vi "KGN Set Concentrations.vi"(6 "Set Values Cluster":T2(array[cluster]), 7 "scaling":dbl, 8 "Fehler (Eingang, kein Fehler)":errorcluster, 9 "Info Cluster":T1, 10 "VISA-Referenz (Eingang)":refnum<visa-resource-name>, 11 "device (Eingang)":u32) -> (0 "Fehler (Ausgang)":errorcluster, 1 "Info Cluster out":T1, 2 "VISA-Referenz (Ausgang)":refnum<visa-resource-name>, 3 "dup device (Ausgang)":u32, 4 "Kommandos gesendet":string)   [LabVIEW 2020, in "Linearisierung v2.lvlib" / "Gasteiler.lvlib" / "HovaCAL_Interface.lvlib" / "KGN.lvlib" / "KGN GUI Set.lvlib"]
uses:
  KGN GUI Set.lvlib
  Controls/Info Cluster.ctl
  set/set.lvlib
  Controls/Controls.lvlib
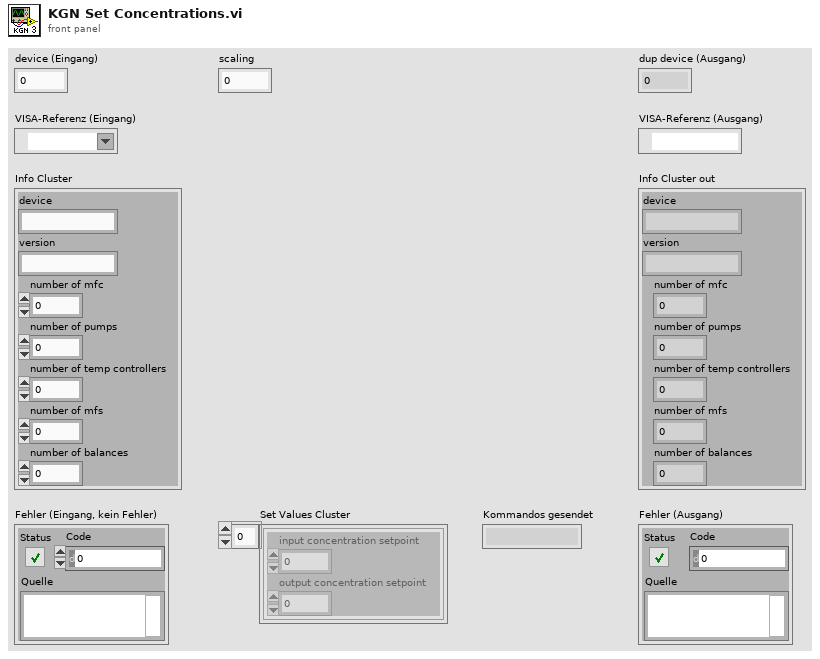
[diagram p1: front panel]
types:
  T1 = typedef "Linearisierung v2.lvlib/Gasteiler.lvlib/HovaCAL_Interface.lvlib/Controls.lvlib/Info Cluster.ctl" = cluster{"device":string, "version":string, "number of mfc":i32, "number of pumps":i32, "number of temp controllers":i32, "number of mfs":i32, "number of balances":i32}
  T2 = cluster{"input concentration setpoint":dbl, "output concentration setpoint":dbl}[]
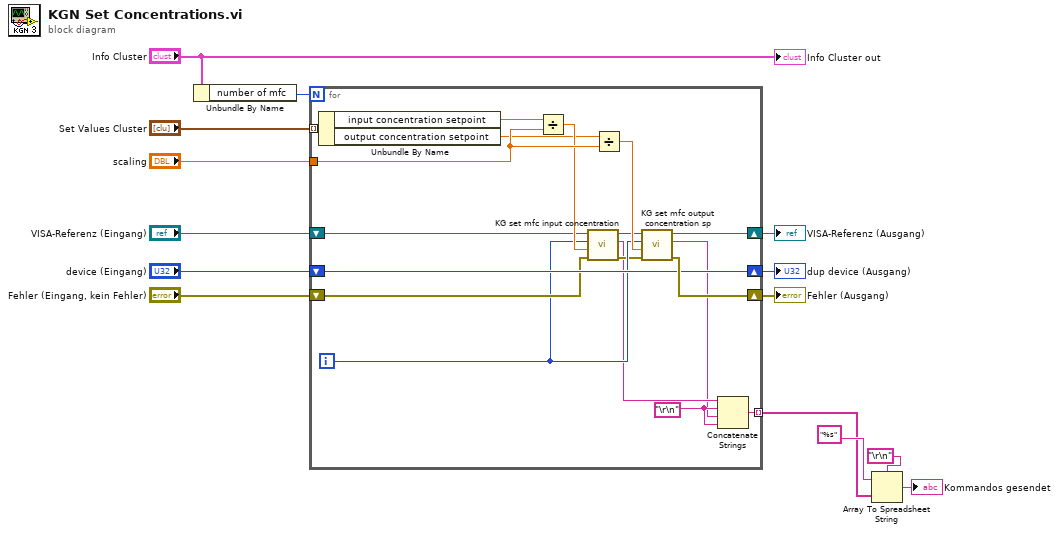
[diagram p0: block diagram]
diagram:
  n1 = Unbundle By Name("Info Cluster") -> ("number of mfc"=w7:i32)
  n2 = for {
    N: w7 -> [_]
    tunnel: "scaling" -> [w32]
    tunnel: "Set Values Cluster" -> [w23] mode=indexing
    shift-right: [w26] -> w12
    shift-left: "device (Eingang)" -> [w26]
    shift-right: [w27] -> w11
    shift-left: "Fehler (Eingang, kein Fehler)" -> [w25]
    shift-right: [w21] -> w5
    shift-left: "VISA-Referenz (Eingang)" -> [w22]
    tunnel: [w15] -> w2 mode=indexing
    i -> [w24]
    w18 = "\r\n"
    n3 = Unbundle By Name(w23) -> ("input concentration setpoint"=w28:dbl, "output concentration setpoint"=w29:dbl)
    n4 = Divide(x=w28, y=w32) -> (x/y=w30:dbl)
    n5 = call "KG set mfc input concentration.vi"("Fehler (Eingang, kein Fehler)"=w25, "concentration"=w30, "mfc"=w24, "VISA-Ressourcenname"=w22) -> ("Fehler (Ausgang)"=w19:errorcluster, "Kommando gesendet"=w17:string, "VISA-Ressourcenname (Ausgang)"=w20:refnum<visa-resource-name>)  [unwired: 5 in]
    n6 = Divide(x=w29, y=w32) -> (x/y=w31:dbl)
    n7 = call "KG set mfc output concentration sp.vi"("Fehler (Eingang, kein Fehler)"=w19, "concentration"=w31, "mfc"=w24, "VISA-Ressourcenname"=w20) -> ("Fehler (Ausgang)"=w27:errorcluster, "kommando gesendet"=w16:string, "VISA-Ressourcenname (Ausgang)"=w21:refnum<visa-resource-name>)  [unwired: 5 in]
    n8 = Concatenate Strings(w17, w18, w16, w18) -> (w15:string)
  }
  "dup device (Ausgang)" <- w12
  "Fehler (Ausgang)" <- w11
  "VISA-Referenz (Ausgang)" <- w5
  n9 = Array To Spreadsheet String(delimiter (Tab)="\r\n", array=w2, 3:"%s" ("Format-String")) -> (spreadsheet string=→"Kommandos gesendet":string)
  "Info Cluster out" <- "Info Cluster"
